vi "Search.vi"(6 "Index in":i32=-1, 7 "Composite Object":refnum<class "CConfig Object.lvclass">, 8 "error in (no error)":errorcluster, 11 "Find Query in":refnum<class "Loop Query.lvclass">) -> (0 "error out":errorcluster, 2 "empty?":bool=TRUE, 3 "Find Query out":refnum<class "Loop Query.lvclass">, 5 "Composite Object":refnum<class "CConfig Object.lvclass">)   [LabVIEW 2013, in "Loop Query.lvclass"]
doc: "Copyright 2018, Carya Automatisering, Wiebe Walstra."
uses:
  Loop Query.lvclass
  CConfig Object.lvclass
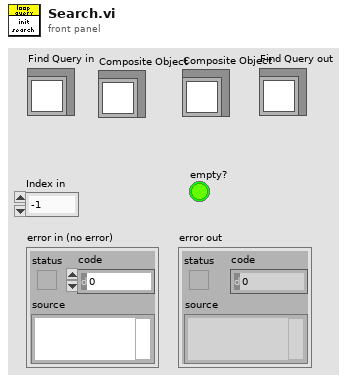
[diagram p1: front panel]
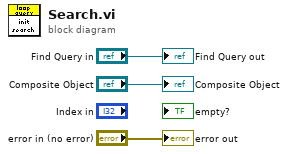
[diagram p0: block diagram]
diagram:
  "error out" <- "error in (no error)"
  "Find Query out" <- "Find Query in"
  "Composite Object" <- "Composite Object"
